vi "TextMark_test.vi"   [LabVIEW 2016]
types:
  T1 = cluster{"VISA Refnum in":refnum<visa-resource-name>, "error in (no error)":errorcluster}
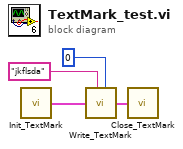
[diagram p0: block diagram]
diagram:
  n1 = call "Init_TextMark.vi"() -> ("TextMark out"=w4:T1)
  n2 = call "Write_TextMark.vi"("text"="jkflsda", "TextMark in"=w4, "type"=0) -> ("TextMark out"=w3:T1)  [unwired: 6 in]
  n3 = call "Close_TextMark.vi"("TextMark in"=w3) -> ()
